vi "Set Default.vi"(11 "ID in":refnum<class "ID.lvclass">) -> (3 "ID out":refnum<class "ID.lvclass">)   [LabVIEW 2022 SP3, in "Conditum.lvlib" / "Columns.lvlib" / "ID.lvclass"]
uses:
  ID.lvclass
  ID.lvclass/ID.ctl
  Type/Type.lvclass
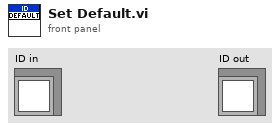
[diagram p1: front panel]
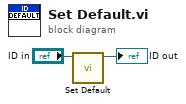
[diagram p0: block diagram]
diagram:
  n1 = call-parent "Set Default.vi"("Type in"="ID in") -> ("Type out"=→"ID out":refnum<class "ID.lvclass">)  [unwired: 10 in]
